vi "MixedGraph.vi"(5 "ZeroedPressure":dbl[][](array[numeric]), 7 "PressureSanity":T3={"PressureErrors"=[], "Plug in titles"=["Good", "AllNegative", "dPTooSmall", "P1smallest", "FailedToReduce", "ExceedMaxCone", "U.LT.0"]}, 8 "OutputErrors2":T4={"PressureErrors"=[], "Plug in titles"=["Good", "AllNegative", "dPTooSmall", "P1smallest", "FailedToReduce", "ExceedMaxCone", "U.LT.0"]}, 9 "RawVmagUVWCone2":dbl[][](array[numeric]), 10 "OutputErrors1":T4={"PressureErrors"=[], "Plug in titles"=["Good", "AllNegative", "dPTooSmall", "P1smallest", "FailedToReduce", "ExceedMaxCone", "U.LT.0"]}, 11 "RawVmagUVWCone1":dbl[][](array[numeric])) -> ()   [LabVIEW 2016]
uses:
  SanityCluster.ctl
  <vilib>/Waveform/DWDTOps.llb/DWDT Boolean Array to Digital.vi
panel:
  in  "Tab Control":enum32{"Graphs", "Inputs"}(tab)
  out "VelHist":T1(graph)
  out "Mixed Signal Graph":T2(graph)
  in  "bins":i32=22
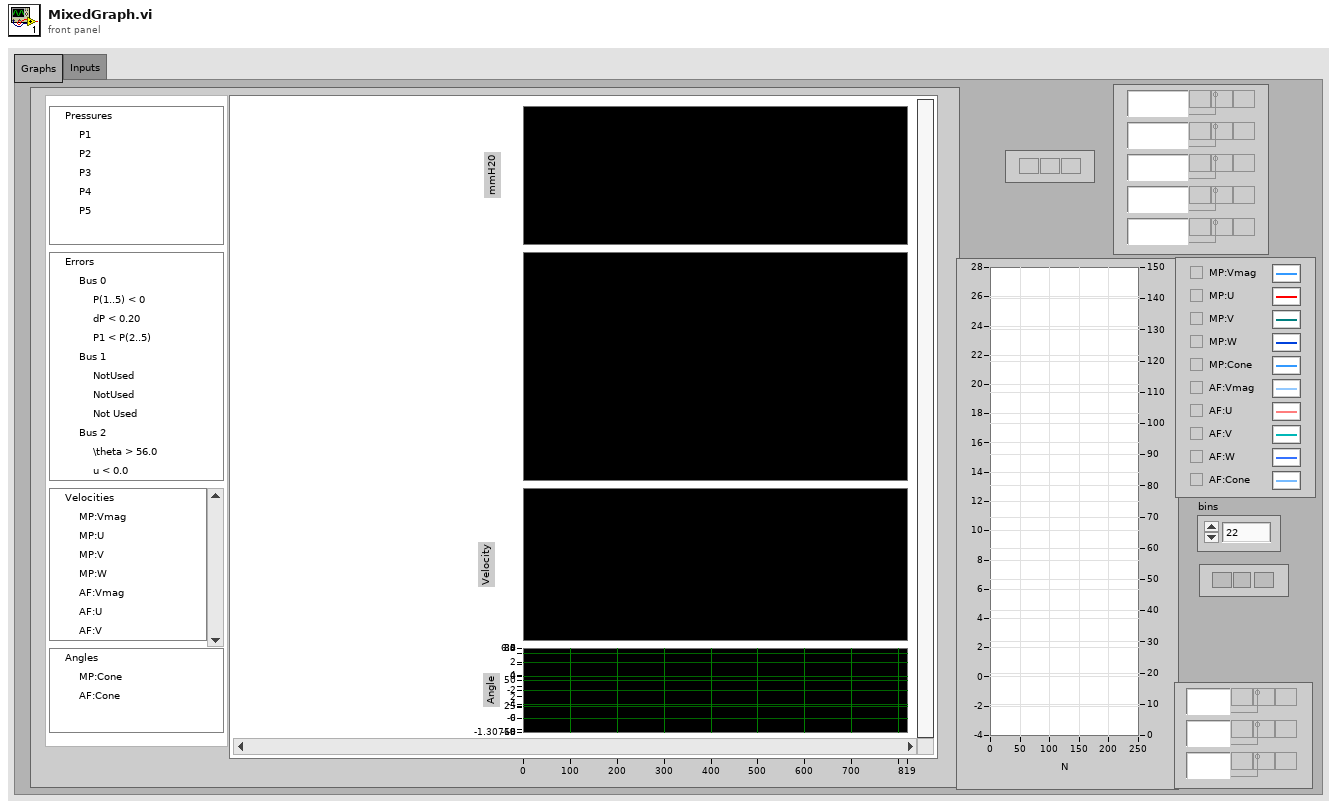
[diagram p1: front panel]
types:
  T1 = cluster{"Histogram: h(x)":i32[], "X Values":dbl[]}[]
  T2 = cluster{"ZeroedPressure":dbl[][], digitalwaveform, digitalwaveform, digitalwaveform, "RawVmagUVWCone1":dbl[][], "RawVmagUVWCone2":dbl[][]}
  T3 = cluster{"PressureErrors":bool[][], "Plug in titles":string[]}
  T4 = typedef "SanityCluster.ctl" = cluster{"PressureErrors":bool[][], "Plug in titles":string[]}
  T5 = cluster{string, "Color Box":u32, "Enum":enum16{"Pressures", "Errors", "Velocity", "Angles"}}[]
  T6 = cluster{string, u32, enum16{"Pressures", "Errors", "Velocity", "Angles"}}[]
  T7 = cluster{string, u32, enum16{"Pressures", "Errors", "Velocity", "Angles"}}
  T8 = cluster{dbl[][], "digital waveform":digitalwaveform, "digital waveform":digitalwaveform, "digital waveform":digitalwaveform, dbl[][], dbl[][]}
  T9 = enum16{"Pressures", "Errors", "Velocity", "Angles"}
  T10 = cluster{"Histogram: h(x)":i32[], "X Values":dbl[]}
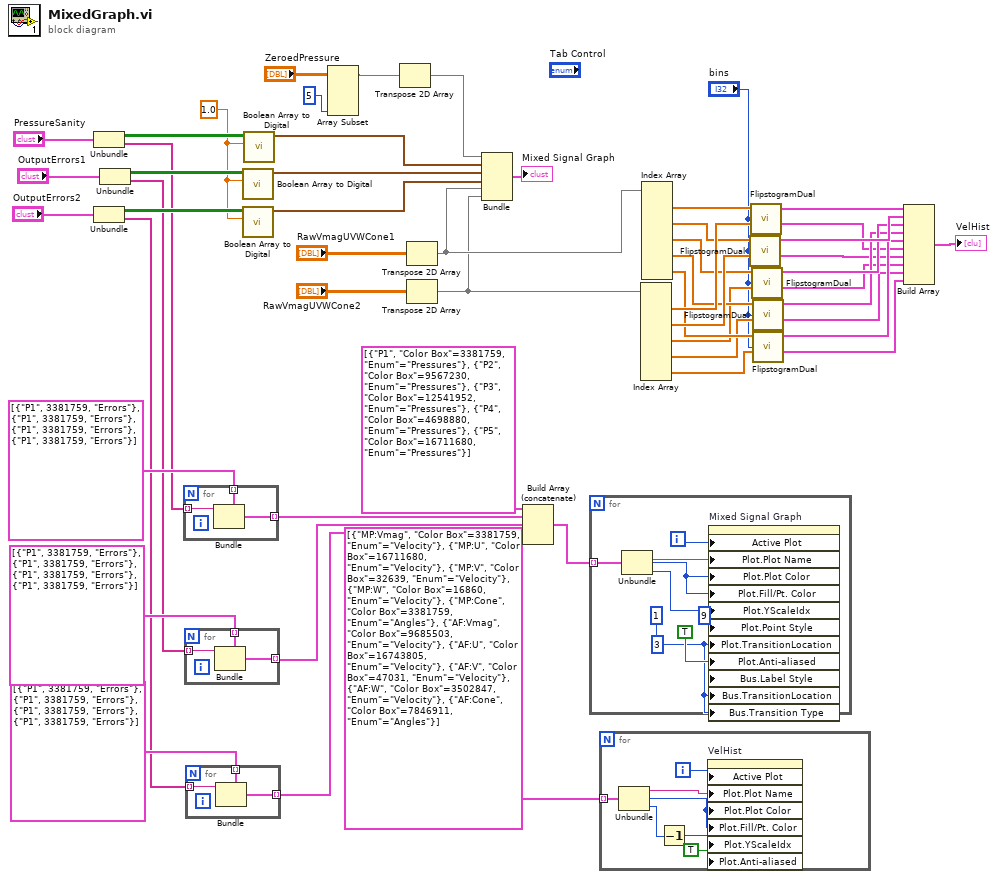
[diagram p0: block diagram]
diagram:
  w34 = 1.0 ("sample rate")
  w24 = T5 [{"MP:Vmag", "Color Box"=3381759, "Enum"=enum."Velocity"}, {"MP:U", "Color Box"=16711680, "Enum"=enum."Velocity"}, {"MP:V", "Color Box"=32639, "Enum"=enum."Velocity"}, {"MP:W", "Color Box"=16860, "Enum"=enum."Velocity"}, {"MP:Cone", "Color Box"=3381759, "Enum"=enum."Angles"}, {"AF:Vmag", "Color Box"=9685503, "Enum"=enum."Velocity"}, {"AF:U", "Color Box"=16743805, "Enum"=enum."Velocity"}, {"AF:V", "Color Box"=47031, "Enum"=enum."Velocity"}, {"AF:W", "Color Box"=3502847, "Enum"=enum."Velocity"}, {"AF:Cone", "Color Box"=7846911, "Enum"=enum."Angles"}] ("Array 2")
  n1 = Unbundle("PressureSanity") -> ("PressureErrors"=w38:bool[][], "Plug in titles"=w31:string[])
  n2 = Unbundle("OutputErrors2") -> ("PressureErrors"=w35:bool[][], "Plug in titles"=w29:string[])
  n3 = Unbundle("OutputErrors1") -> ("PressureErrors"=w36:bool[][], "Plug in titles"=w30:string[])
  n4 = for {
    tunnel: w31 -> [w56] mode=indexing
    tunnel: T6 [{"P1", 3381759, enum."Errors"}, {"P1", 3381759, enum."Errors"}, {"P1", 3381759, enum."Errors"}, {"P1", 3381759, enum."Errors"}] -> [w55] mode=indexing
    tunnel: [w54] -> w41 mode=indexing
    n5 = Bundle(cluster=w55, w56) -> (w54:T7)  [unwired: 2 in]
  }
  n6 = for {
    tunnel: T6 [{"P1", 3381759, enum."Errors"}, {"P1", 3381759, enum."Errors"}, {"P1", 3381759, enum."Errors"}, {"P1", 3381759, enum."Errors"}] -> [w59] mode=indexing
    tunnel: [w58] -> w40 mode=indexing
    tunnel: w30 -> [w57] mode=indexing
    n7 = Bundle(cluster=w59, w57) -> (w58:T7)  [unwired: 2 in]
  }
  n8 = for {
    tunnel: T6 [{"P1", 3381759, enum."Errors"}, {"P1", 3381759, enum."Errors"}, {"P1", 3381759, enum."Errors"}, {"P1", 3381759, enum."Errors"}] -> [w62] mode=indexing
    tunnel: [w61] -> w39 mode=indexing
    tunnel: w29 -> [w60] mode=indexing
    n9 = Bundle(cluster=w62, w60) -> (w61:T7)  [unwired: 2 in]
  }
  n10 = call-poly <vilib>:"Boolean Array to Digital.vi"("sample rate"=w34, "boolean array"=w36) -> ("digital waveform"=w33:digitalwaveform)  [unwired: 8 in, 1 out]
  n11 = call-poly <vilib>:"Boolean Array to Digital.vi"("sample rate"=w34, "boolean array"=w35) -> ("digital waveform"=w32:digitalwaveform)  [unwired: 8 in, 1 out]
  n12 = call-poly <vilib>:"Boolean Array to Digital.vi"("sample rate"=w34, "boolean array"=w38) -> ("digital waveform"=w37:digitalwaveform)  [unwired: 8 in, 1 out]
  n13 = Array Subset(array="ZeroedPressure", length (col)=5 ("length")) -> (w2:dbl[][])  [unwired: 3 in]
  n14 = Transpose 2D Array(2D array=w2) -> (transposed array=w48:dbl[][])
  n15 = Transpose 2D Array(2D array="RawVmagUVWCone1") -> (transposed array=w27:dbl[][])
  n16 = Transpose 2D Array(2D array="RawVmagUVWCone2") -> (transposed array=w25:dbl[][])
  n17 = Bundle(w48, "digital waveform"=w37, "digital waveform"=w33, "digital waveform"=w32, w27, w25) -> (→"Mixed Signal Graph":T8)  [unwired: 1 in]
  n18 = Build Array (concatenate)(T5 [{"P1", "Color Box"=3381759, "Enum"=enum."Pressures"}, {"P2", "Color Box"=9567230, "Enum"=enum."Pressures"}, {"P3", "Color Box"=12541952, "Enum"=enum."Pressures"}, {"P4", "Color Box"=4698880, "Enum"=enum."Pressures"}, {"P5", "Color Box"=16711680, "Enum"=enum."Pressures"}] ("Array 2"), w41, w40, w39, w24) -> (w44:T5)
  n19 = for {
    tunnel: w44 -> [w71] mode=indexing
    i -> [w69]
    w65 = u8 1 ("Bus.Digital Transition Location")
    n20 = Unbundle(w71) -> (w70:string, "Color Box"=w63:u32, "Enum"=w68:T9)
    n21 = property on="Mixed Signal Graph" class="MixedGraph (strict)"("Active Plot"=w69, "Plot.Plot Name"=w70, "Plot.Plot Color"=w63, "Plot.Fill/Pt. Color"=w63, "Plot.YScaleIdx"=w68, "Plot.Point Style"=u8 9, "Plot.TransitionLocation"=w65, "Plot.Anti-aliased"=TRUE, "Bus.Label Style"=u8 3 ("Bus.Label Format"), "Bus.TransitionLocation"=w65, "Bus.Transition Type"=w65) -> ()  [unwired: 2 in, 2 out]
  }
  n22 = for {
    tunnel: w24 -> [w77] mode=indexing
    i -> [w78]
    n23 = Unbundle(w77) -> (w76:string, "Color Box"=w75:u32, "Enum"=w73:T9)
    n24 = Decrement(x=w73) -> (x-1=w72:T9)
    n25 = property on="VelHist" class="XYGraph (strict)"("Active Plot"=w78, "Plot.Plot Name"=w76, "Plot.Plot Color"=w75, "Plot.Fill/Pt. Color"=w75, "Plot.YScaleIdx"=w72, "Plot.Anti-aliased"=TRUE) -> ()  [unwired: 2 in, 2 out]
  }
  n26 = Index Array(array=w25) -> (element #1=w21:dbl[], element #2=w17:dbl[], element #3=w13:dbl[], element #4=w12:dbl[], element #5=w20:dbl[])  [unwired: 10 in]
  n27 = Index Array(array=w27) -> (element #1=w23:dbl[], element #2=w18:dbl[], element #3=w16:dbl[], element #4=w15:dbl[], element #5=w14:dbl[])  [unwired: 10 in]
  n28 = call "FlipstogramDual.vi"("intervals"="bins", "Array2"=w17, "Array1"=w18) -> ("Flipst2"=w5:T10, "Flipst1"=w11:T10)  [unwired: 4 in]
  n29 = call "FlipstogramDual.vi"("intervals"="bins", "Array2"=w21, "Array1"=w23) -> ("Flipst2"=w4:T10, "Flipst1"=w22:T10)  [unwired: 4 in]
  n30 = call "FlipstogramDual.vi"("intervals"="bins", "Array2"=w13, "Array1"=w16) -> ("Flipst2"=w6:T10, "Flipst1"=w10:T10)  [unwired: 4 in]
  n31 = call "FlipstogramDual.vi"("intervals"="bins", "Array2"=w12, "Array1"=w15) -> ("Flipst2"=w7:T10, "Flipst1"=w9:T10)  [unwired: 4 in]
  n32 = call "FlipstogramDual.vi"("intervals"="bins", "Array2"=w20, "Array1"=w14) -> ("Flipst2"=w19:T10, "Flipst1"=w8:T10)  [unwired: 4 in]
  n33 = Build Array(w22, w11, w10, w9, w8, w4, w5, w6, w7, w19) -> (→"VelHist":T1)
